vi "CNR abx reweighted (Pearson option).vi"(0 "parameters":dbl[](array[numeric]), 1 "model function":T4, 5 "method":T2 items=["Least Square", "Least Absolute Residual", "Bisquare"], 7 "scale factors":dbl[](array[numeric]), 9 "output control":T3={"model function"=TRUE, "gradient"=TRUE}, 11 "error in (no error)":errorcluster, 12 "Y":dbl[](array[numeric]), 13 "X":dbl[](array[numeric]), 14 "Weight":dbl[](array[numeric])) -> (2 "Jacobian":T1, 3 "number of function calls":i32, 4 "Hessian":T1, 6 "gradient":dbl[](array[numeric]), 8 "best fit":dbl[](array[numeric]), 10 "chiSqr":dbl, 15 "error out":errorcluster)   [LabVIEW 2021, in "Fits.lvlib"]
uses:
  Fits.lvlib
  <vilib>/Analysis/Matrix/Datatypes/RealMatrix.ctl
  <vilib>/gmath/NumericalOptimization/LM model function.ctl
  <vilib>/gmath/NumericalOptimization/LM model function reference.ctl
  <vilib>/gmath/NumericalOptimization/LM_output select.ctl
  <vilib>/Analysis/6fits.llb/Curve Fitting Criteria.ctl
  <vilib>/Analysis/baseanly.llb/Real Dot Product.vi
  <vilib>/Analysis/baseanly.llb/A x Vector.vi
  <vilib>/Analysis/baseanly.llb/Real A x B.vi
  <vilib>/gmath/NI_Gmath.lvlib
  <vilib>/Analysis/NI_AALBase.lvlib
  <vilib>/Analysis/Matrix/NI_Matrix.lvlib
  <vilib>/Analysis/NI_AALPro.lvlib
panel:
  # "Lev-Mar\nabx"
  # "see the License on the block diagram (Ctrl+E or Window:Show Block Diagram)"
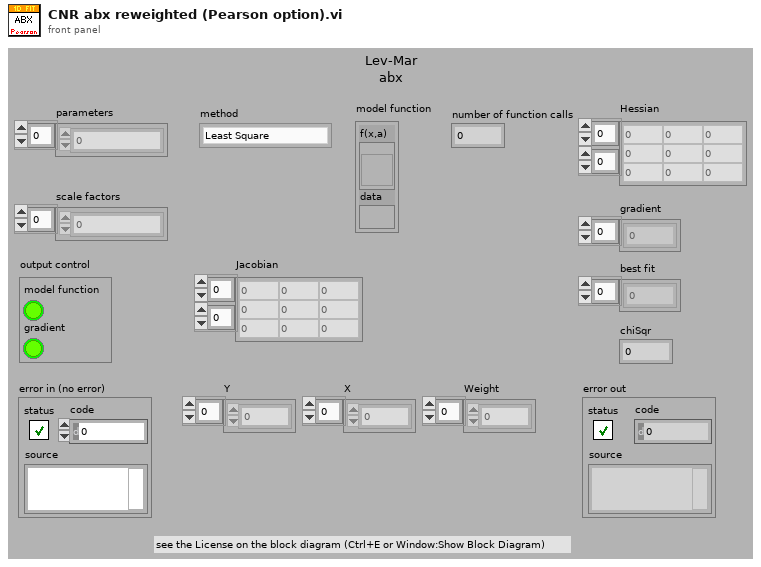
[diagram p1: front panel]
types:
  T1 = typedef "NI_Matrix.lvlib/RealMatrix.ctl" = dbl[][]
  T2 = typedef "NI_AALPro.lvlib/Curve Fitting Criteria.ctl" = u16
  T3 = typedef "NI_Gmath.lvlib/LM_output select.ctl" = cluster{"model function":bool, "gradient":bool}
  T4 = typedef "NI_Gmath.lvlib/LM model function.ctl" = cluster{"f(x,a)":T5, "data":variant}
  T5 = typedef "NI_Gmath.lvlib/LM model function reference.ctl" = refnum<vi>
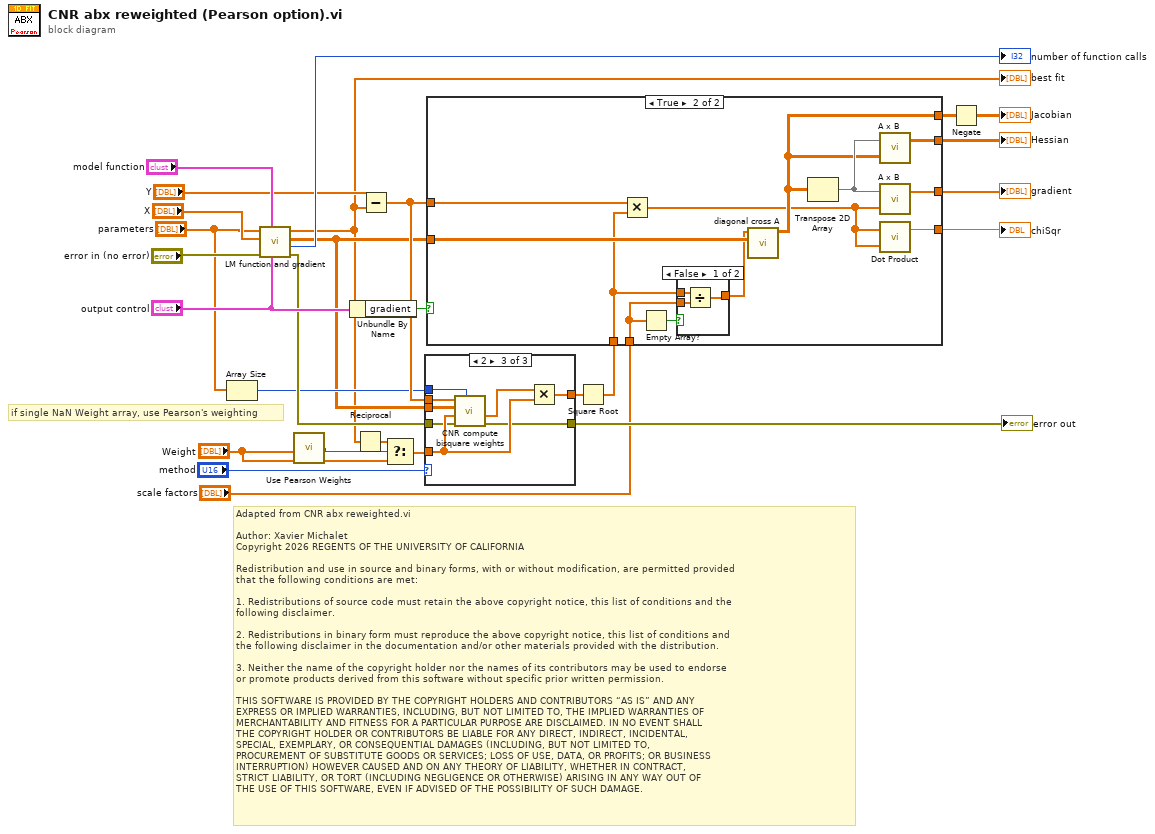
[diagram p0: block diagram]
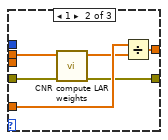
[diagram p3: hidden frame]
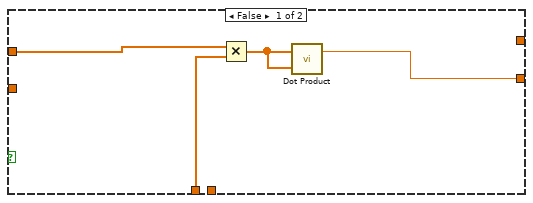
[diagram p4: hidden frame]
diagram:
  # "if single NaN Weight array, use Pearson's weighting"
  # "Adapted from CNR abx reweighted.vi\n\nAuthor: Xavier Michalet\nCopyright 2026 REGENTS OF THE UNIVERSITY OF CALIFORNIA\n\nRedistribution and use in source and binary forms, with or without modification, are permitted provided\nthat the following conditions are met:\n\n1. Redistributions of source code must retain the above copyright notice, this list of conditions and the\nfollowing disclaimer.\n\n2. Redistributions in binary form must reproduce the above copyright notice, this list of conditions and\nthe following disclaimer in the documentation and/or other materials provided with the distribution.\n\n3. Neither the name of the copyright holder nor the names of its contributors may be used to endorse \nor promote products derived from this software without specific prior written permission.\n\nTHIS SOFTWARE IS PROVIDED BY THE COPYRIGHT HOLDERS AND CONTRIBUTORS “AS IS” AND ANY \nEXPRESS OR IMPLIED WARRANTIES, INCLUDING, BUT NOT LIMITED TO, THE IMPLIED WARRANTIES OF\nMERCHANTABILITY AND FITNESS FOR A PARTICULAR PURPOSE ARE DISCLAIMED. IN NO EVENT SHALL\nTHE COPYRIGHT HOLDER OR CONTRIBUTORS BE LIABLE FOR ANY DIRECT, INDIRECT, INCIDENTAL, \nSPECIAL, EXEMPLARY, OR CONSEQUENTIAL DAMAGES (INCLUDING, BUT NOT LIMITED TO, \nPROCUREMENT OF SUBSTITUTE GOODS OR SERVICES; LOSS OF USE, DATA, OR PROFITS; OR BUSINESS\nINTERRUPTION) HOWEVER CAUSED AND ON ANY THEORY OF LIABILITY, WHETHER IN CONTRACT, \nSTRICT LIABILITY, OR TORT (INCLUDING NEGLIGENCE OR OTHERWISE) ARISING IN ANY WAY OUT OF\nTHE USE OF THIS SOFTWARE, EVEN IF ADVISED OF THE POSSIBILITY OF SUCH DAMAGE."
  n1 = Array Size(array="parameters") -> (size(s)=w13:i32)
  n2 = call <vilib>:"LM function and gradient.vi"("output control"="output control", "model function"="model function", "error in (no error)"="error in (no error)", "X"="X", "a"="parameters") -> ("error out"=w21:errorcluster, "number of function calls"=→"number of function calls":i32, "gradient"=w8:dbl[][], "f(X)"=w4:dbl[])  [unwired: 3 out]
  "best fit" <- w4
  n3 = call "Use Pearson Weights.vi"("Weight"="Weight") -> ("Use Pearson Weight"=w1:bool)
  n4 = Unbundle By Name("output control") -> ("gradient"=w23:bool)
  n5 = Reciprocal(x=w4) -> (1/x=w3:dbl[])
  n6 = Subtract(x="Y", y=w4) -> (x-y=w14:dbl[])
  n7 = Select(t=w3, s=w1, f="Weight") -> (s? t:f=w5:dbl[])
  n8 = case shown="2" "method" {
    tunnel: w8 -> [_ _ w43]
    tunnel: [w29 w34 w42] -> w10
    tunnel: w5 -> [w29 w35 w41]
    tunnel: [w28 w30 w40] -> w17
    tunnel: w21 -> [w28 w31 w39]
    tunnel: w14 -> [_ w33 w38]
    tunnel: w13 -> [_ _ w36]
    frame 0, Default {
    }
    frame 1 {
      n9 = call <vilib>:"CNR compute LAR weights.vi"("error in (no error)"=w31, "residuals"=w33) -> ("error out"=w30:errorcluster, "LAR weights"=w32:dbl[])  [unwired: 8 out]
      n10 = Divide(x=w35, y=w32) -> (x/y=w34:dbl[])
    }
    frame 2 {
      n11 = call <vilib>:"CNR compute bisquare weights.vi"("number of parameters"=w36, "error in (no error)"=w39, "weight"=w41, "J"=w43, "raw residuals"=w38) -> ("error out"=w40:errorcluster, "weights"=w37:dbl[])  [unwired: 5 out]
      n12 = Multiply(x=w37, y=w41) -> (x*y=w42:dbl[])
    }
  }
  "error out" <- w17
  n13 = Square Root(x=w10) -> (sqrt(x)=w11:dbl[])
  n14 = case shown="True" w23 {
    tunnel: [_ w49] -> w18
    tunnel: [_ w50] -> w6
    tunnel: [w44 w59] -> w27
    tunnel: w8 -> [_ w58]
    tunnel: w11 -> [w47 w55]
    tunnel: w14 -> [w46 w57]
    tunnel: "scale factors" -> [_ w53]
    tunnel: [_ w51] -> w7
    frame False {
      n15 = Multiply(x=w46, y=w47) -> (x*y=w45:dbl[])
      n16 = call-poly <vilib>:"Dot Product.vi"("Y Vector"=w45, "X Vector"=w45) -> ("X * Y"=w44:dbl)  [unwired: 1 out]
    }
    frame True {
      n17 = Multiply(x=w57, y=w55) -> (x*y=w48:dbl[])
      n18 = Empty Array?(array=w53) -> (empty?=w52:bool)
      n19 = case shown="False" w52 {
        tunnel: w55 -> [w62 w63]
        tunnel: w53 -> [w61 _]
        tunnel: [w60 w63] -> w54
        frame False {
          n20 = Divide(x=w62, y=w61) -> (x/y=w60:dbl[])
        }
        frame True {
        }
      }
      n21 = call <vilib>:"diagonal cross A.vi"("A"=w58, "diagonal"=w54) -> ("diagonalxA"=w51:T1)  [unwired: 9 out]
      n22 = Transpose 2D Array(2D array=w51) -> (transposed array=w56:T1)
      n23 = call-poly <vilib>:"A x B.vi"("B"=w51, "A"=w56) -> ("A x B"=w50:T1)  [unwired: 1 out]
      n24 = call-poly <vilib>:"A x B.vi"("Vector"=w48, "A"=w56) -> ("A x Vector"=w49:dbl[])  [unwired: 1 out]
      n25 = call-poly <vilib>:"Dot Product.vi"("Y Vector"=w48, "X Vector"=w48) -> ("X * Y"=w59:dbl)  [unwired: 1 out]
    }
  }
  "Hessian" <- w6
  "gradient" <- w18
  "chiSqr" <- w27
  n26 = Negate(x=w7) -> (-x=→"Jacobian":T1)
